vi "from string.vi"(8 "error in":errorcluster, 9 "data":string, 10 "version":string, 11 "EthernetIP configuration in":refnum<class "EIP Tags Configuration.lvclass">) -> (0 "error out":errorcluster, 3 "EthernetIP configuration out":refnum<class "EIP Tags Configuration.lvclass">)   [LabVIEW 2013, in "EIP Tags Configuration.lvclass"]
doc: "Provides an interface for loading a module configuration from a file or other serialized data source. It is recommended that all children of this class store data in two sets--data required for its own initialization, and any data required for parent initialization--and that each implementation uses the <b>Call Parent Method</b> primitive to de-serialize parent information. As a result, it is expected that every module configuration class calls <b>component configuration.lvclass:From String.vi</b>."
uses:
  EIP Tags Configuration.lvclass
  eip tag definition.ctl
  eip tag types.ctl
  channel/EIP Tags Channel.lvclass
  <vilib>/NI/Tag Bus Module Framework/module configuration/TBM module configuration.lvclass
  EIP Tags Configuration.lvclass/EIP Tags Configuration.ctl
  <vilib>/NI/Configuration Framework/serializable configuration/NISE_CEF_serializable configuration.lvclass
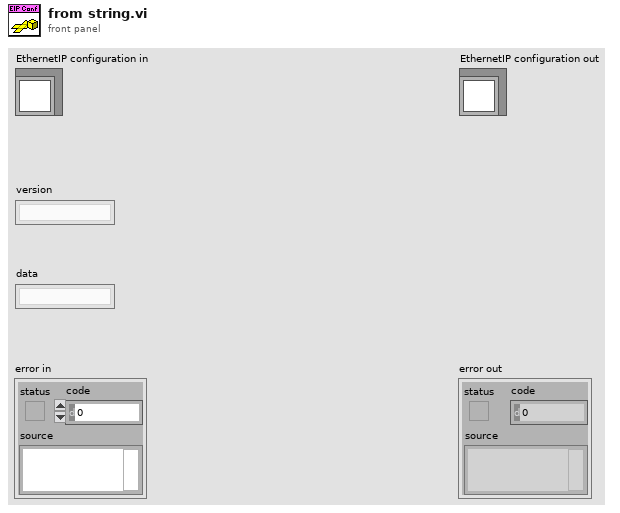
[diagram p1: front panel]
types:
  T1 = typedef "EIP Tags Configuration.lvclass/eip tag definition.ctl" = cluster{"eip tag types":T2, "unique tag name":string, "Number of Elements":u32}
  T2 = typedef "EIP Tags Configuration.lvclass/eip tag types.ctl" = enum16{"SINT", "INT", "DINT", "REAL", "BOOL", "STRING"}
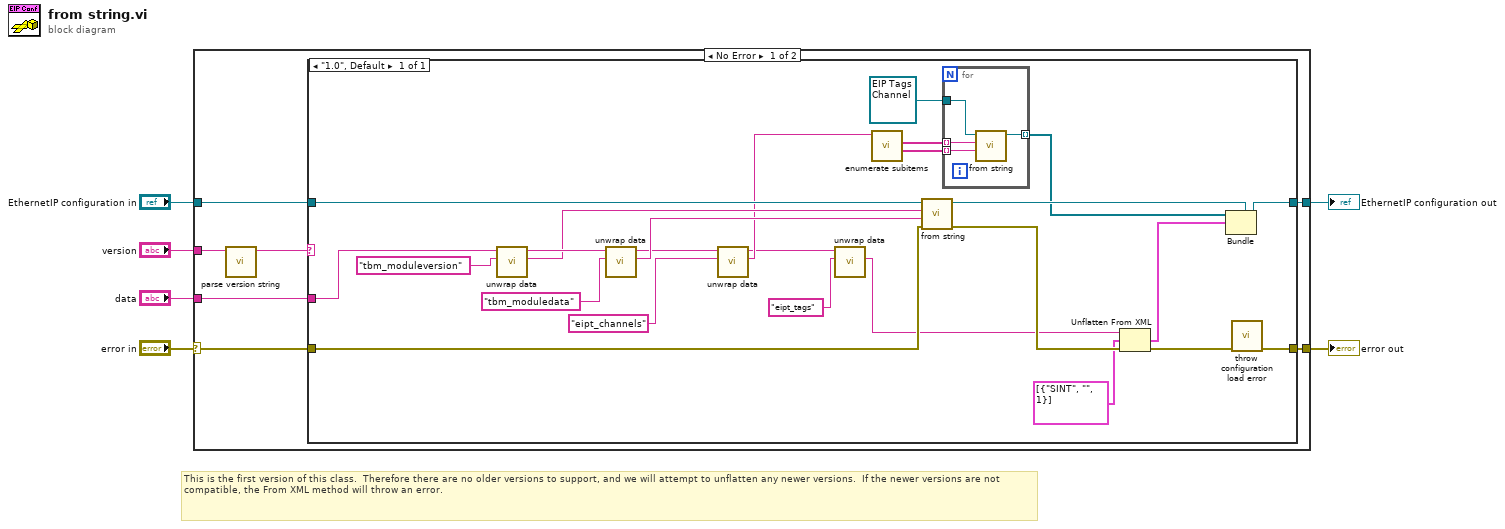
[diagram p0: block diagram]
diagram:
  # "This is the first version of this class.  Therefore there are no older versions to support, and we will attempt to unflatten any newer versions.  If the newer versions are not compatible, the From XML method will throw an error."
  n1 = case shown="No Error" "error in" {
    selector: "error in" -> [w7 w44]
    tunnel: "data" -> [w13 _]
    tunnel: "EthernetIP configuration in" -> [w12 w43]
    tunnel: [w11 w43] -> w5
    tunnel: [w10 w44] -> w4
    tunnel: "version" -> [w9 _]
    frame No Error {
      n2 = call <vilib>:"parse version string.vi"("full version"=w9) -> ("major.minor version"=w8:string)  [unwired: 7 in, 3 out]
      n3 = case shown="\"1.0\", Default" w8 {
        tunnel: w13 -> [w34]
        tunnel: w7 -> [w33]
        tunnel: w12 -> [w38]
        tunnel: [w28] -> w11
        tunnel: [w36] -> w10
        frame "1.0", Default {
          n4 = call <vilib>:"unwrap data.vi"("identifier"="tbm_moduleversion" ("additional identifier"), "data to unwrap"=w34) -> ("unwrapped data"=w29:string, "remaining string"=w35:string)  [unwired: 8 in]
          n5 = call <vilib>:"unwrap data.vi"("identifier"="tbm_moduledata" ("additional identifier"), "data to unwrap"=w35) -> ("unwrapped data"=w31:string, "remaining string"=w27:string)  [unwired: 8 in]
          n6 = call <vilib>:"unwrap data.vi"("identifier"="eipt_channels" ("additional identifier"), "data to unwrap"=w27) -> ("unwrapped data"=w26:string, "remaining string"=w18:string)  [unwired: 8 in]
          n7 = call <vilib>:"unwrap data.vi"("identifier"="eipt_tags" ("additional identifier"), "data to unwrap"=w18) -> ("unwrapped data"=w17:string)  [unwired: 8 in, 1 out]
          n8 = call <vilib>:"enumerate subitems.vi"("data to enumerate"=w26) -> ("associated data"=w24:string[], "discovered subitems"=w25:string[])  [unwired: 8 in, 1 out]
          n9 = call-parent "from string.vi"("error in"=w33, "data"=w31, "version"=w29, "module configuration in"=w38) -> ("error out"=w22:errorcluster, "module configuration out"=w37:refnum<class "EIP Tags Configuration.lvclass">)  [unwired: 6 in]
          n10 = for {
            tunnel: w25 -> [w42] mode=indexing
            tunnel: w24 -> [w41] mode=indexing
            tunnel: [w40] -> w23 mode=indexing
            tunnel: refnum<class "EIP Tags Channel.lvclass"> refnum ("EIP Tags Channel.lvclass") -> [w39]
            n11 = call-dynamic "from string.vi"("channel data"=w41, "identifier"=w42, "channel in"=w39) -> ("channel out"=w40:refnum<class "EIP Tags Channel.lvclass">)  [unwired: 7 in, 1 out]
          }
          n12 = Unflatten From XML(xml string=w17, type=T1[] [{"eip tag types"=enum."SINT", "unique tag name"="", "Number of Elements"=1}] ("assemblies"), error in (no error)=w22) -> (value=w19:T1[], error out=w21:errorcluster)
          n13 = Bundle(cluster=w37, w23, w19) -> (w28:refnum<class "EIP Tags Configuration.lvclass">)  [unwired: 1 in]
          n14 = call <vilib>:"throw configuration load error.vi"("error in"=w21) -> ("error out"=w36:errorcluster)  [unwired: 10 in]
        }
      }
    }
    frame Error {
    }
  }
  "error out" <- w4
  "EthernetIP configuration out" <- w5
